vi "Ctor.vi"(8 "error in (no error)":errorcluster) -> (0 "error out":errorcluster, 3 "SOL-Server out":refnum<class "SOL-Server.lvclass">)   [LabVIEW 2020, in "Summer of LabVIEW.lvlib" / "SOL-Server.lvclass"]
uses:
  SOL-Server.lvclass
  SOL-Server.lvclass/SOL-Server.ctl
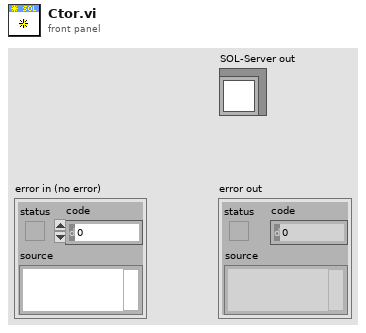
[diagram p1: front panel]
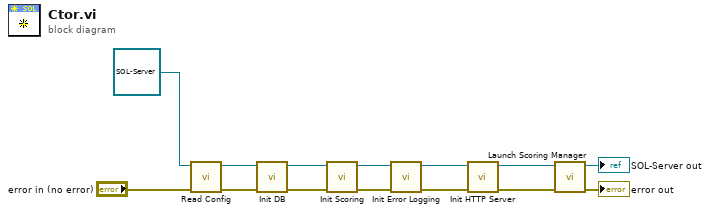
[diagram p0: block diagram]
diagram:
  n1 = call "Read Config.vi"("error in (no error)"="error in (no error)", "SOL-Server in"=refnum<class "SOL-Server.lvclass"> refnum ("SOL-Server out")) -> ("error out"=w8:errorcluster, "SOL-Server out"=w7:refnum<class "SOL-Server.lvclass">)  [unwired: 8 in]
  n2 = call "Init DB.vi"("error in (no error)"=w8, "SOL-Server in"=w7) -> ("error out"=w9:errorcluster, "SOL-Server out"=w10:refnum<class "SOL-Server.lvclass">)  [unwired: 8 in]
  n3 = call "Init Scoring.vi"("error in (no error)"=w9, "SOL-Server in"=w10) -> ("error out"=w3:errorcluster, "SOL-Server out"=w4:refnum<class "SOL-Server.lvclass">)  [unwired: 8 in]
  n4 = call "Init Error Logging.vi"("error in (no error)"=w3, "SOL-Server in"=w4) -> ("error out"=w2:errorcluster, "SOL-Server out"=w1:refnum<class "SOL-Server.lvclass">)  [unwired: 8 in]
  n5 = call "Init HTTP Server.vi"("error in (no error)"=w2, "SOL-Server in"=w1) -> ("error out"=w13:errorcluster, "SOL-Server out"=w14:refnum<class "SOL-Server.lvclass">)  [unwired: 8 in]
  n6 = call "Launch Scoring Manager.vi"("error in (no error)"=w13, "SOL-Server in"=w14) -> ("error out"=→"error out":errorcluster, "SOL-Server out"=→"SOL-Server out":refnum<class "SOL-Server.lvclass">)  [unwired: 8 in]
